vi "Format to Technique Parameter (Depreciated).vi"(0 "Potentiostat Galvanostat in":refnum<class "Potentiostat Galvanostat.lvclass">, 5 "Parameter Label":string, 7 "Parameter":variant, 9 "Parameter Index":i32, 11 "error in (no error)":errorcluster) -> (4 "Potentiostat Galvanostat out":refnum<class "Potentiostat Galvanostat.lvclass">, 8 "Technique Parameter":T1 {"Parameter Type" items=["I32 (Long)", "BOOL (Boolean)", "SGL (Single Precision)"]}, 15 "error out":errorcluster)   [LabVIEW 2018, in "Potentiostat Galvanostat.lvclass"]
doc: "This function tests the communication speed between the library and the selected channel. \nNOTE: This function is for advanced user only."
uses:
  Potentiostat Galvanostat.lvclass
  Controls/Technique Parameter.ctl
  Controls/Parameter Type.ctl
  Controls/Error Codes.ctl
  Potentiostat Galvanostat.lvclass/Potentiostat Galvanostat.ctl
  BL_GetErrorMsg.vi
  <vilib>/Utility/error.llb/Error Cluster From Error Code.vi
  <vilib>/Utility/Data Type/NI_Data Type.lvlib
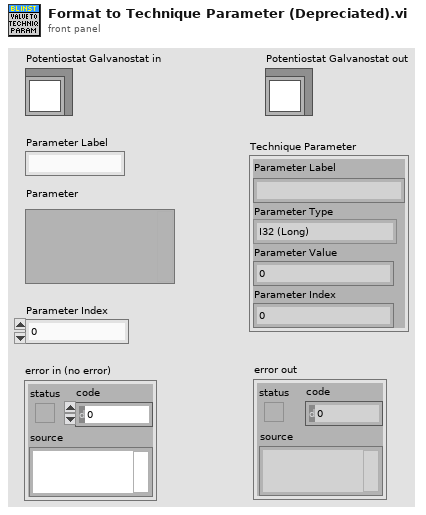
[diagram p1: front panel]
types:
  T1 = typedef "Potentiostat Galvanostat.lvclass/Technique Parameter.ctl" = cluster{"Parameter Label":string, "Parameter Type":T2, "Parameter Value":i32, "Parameter Index":i32}
  T2 = typedef "Potentiostat Galvanostat.lvclass/Parameter Type.ctl" = i32
  T3 = typedef "NI_Data Type.lvlib/Data Type.ctl" = enum8{"Invalid Type", "Void", "I8", "I16", "I32", "I64", "U8", "U16", "U32", "U64", "Single Float", "Double Float", "Extended Float", "Single Complex", "Double Complex", "Extended Complex", "Enum U8", "Enum U16", "Enum U32", "Enum U64", "Single Float With Unit", "Double Float With Unit", "Extended Float With Unit", "Single Complex with Unit", "Double Complex with Unit", "Extended Complex with Unit", "Boolean", "String", "Path", "Picture", "Tag", "Array", "Cluster", "Variant", "LV Variant", "Waveform", "Timestamp", "Digital Waveform", "Digital Data", "ExpressData", "Refnum", "External Data", "VI", "Poly VI", "LabVIEW Class Instance", "Fixed Point"}
  T4 = typedef "Potentiostat Galvanostat.lvclass/Error Codes.ctl" = i32
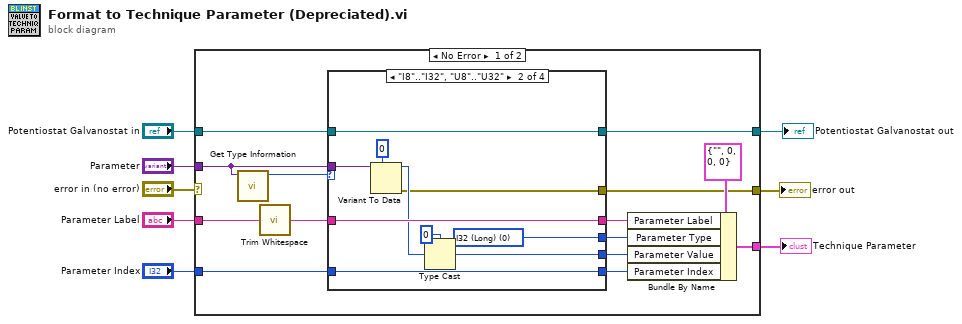
[diagram p0: block diagram]
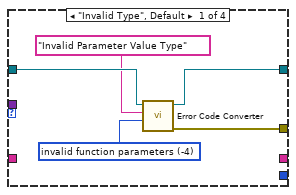
[diagram p2: hidden frame]
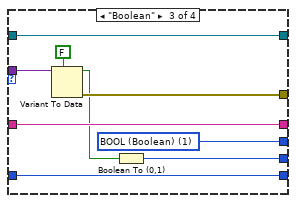
[diagram p3: hidden frame]
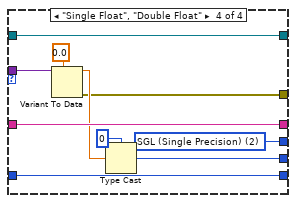
[diagram p4: hidden frame]
diagram:
  n1 = case shown="No Error" "error in (no error)" {
    selector: "error in (no error)" -> [_ w57]
    tunnel: "Parameter" -> [w10 _]
    tunnel: "Potentiostat Galvanostat in" -> [w22 w58]
    tunnel: "Parameter Label" -> [w12 _]
    tunnel: "Parameter Index" -> [w21 _]
    tunnel: [w20 _] -> w4
    tunnel: [w14 w57] -> w3
    tunnel: [w13 w58] -> w2
    frame No Error {
      n2 = call <vilib>:"Get Type Information.vi"("Variant"=w10) -> ("Type"=w9:T3)  [unwired: 6 in, 4 out]
      n3 = call <vilib>:"Trim Whitespace.vi"("string"=w12) -> ("trimmed string"=w11:string)  [unwired: 1 in]
      n4 = case shown="\"I8\"..\"I32\", \"U8\"..\"U32\"" w9 {
        tunnel: w10 -> [_ w37 w46 w56]
        tunnel: w22 -> [w27 w28 w40 w47]
        tunnel: [w26 w28 w40 w47] -> w13
        tunnel: [w25 w29 w41 w48] -> w14
        tunnel: w11 -> [_ w35 w44 w54]
        tunnel: w21 -> [_ w34 w43 w53]
        tunnel: [_ w35 w44 w54] -> w18
        tunnel: [_ w30 w42 w49] -> w17
        tunnel: [_ w33 w39 w52] -> w16
        tunnel: [_ w34 w43 w53] -> w15
        frame "Invalid Type", Default {
          w23 = T4 -4 items=["No Error"=0, "no instrument connected"=-1, "connection in progress"=-2, "selected channel(s) unplugged"=-3, "invalid function parameters"=-4, "selected file does not exist"=-5, "function failed"=-6, "no channel selected"=-7, "invalid instrument configuration"=-8, "EC-Lab firmware loaded on the instrument"=-9, "library not correctly loaded in memory"=-10, "USB library not correctly loaded in memory"=-11, "function of the library already in progress"=-12, "selected channel(s) already used"=-13, "device not allowed"=-14, "Invalid update function parameters"=-15, "internal instrument communication failed"=-101, "too many data to transfer from the instrument (device error)"=-102, "selected channel(s) unplugged (device error)"=-103, "instrument response error"=-104, "invalid message size"=-105] ("Error Code")
          n5 = call "Error Code Converter.vi"("Error Code"=w23, "Additional Description"="Invalid Parameter Value Type", "Potentiostat Galvanostat in"=w27) -> ("error out"=w25:errorcluster, "Potentiostat Galvanostat out"=w26:refnum<class "Potentiostat Galvanostat.lvclass">)  [unwired: 7 in]
        }
        frame "I8".."I32", "U8".."U32" {
          w30 = T2 0 items=["I32 (Long)", "BOOL (Boolean)", "SGL (Single Precision)"] ("Parameter Type")
          n6 = Variant To Data(type=0, Variant=w37) -> (data=w31:i32, error out=w29:errorcluster)  [unwired: 1 in]
          n7 = Type Cast(type=0, x=w31) -> (*(type *) &x=w33:i32)
        }
        frame "Boolean" {
          w42 = T2 1 items=["I32 (Long)", "BOOL (Boolean)", "SGL (Single Precision)"] ("Parameter Type")
          n8 = Variant To Data(type=FALSE, Variant=w46) -> (data=w38:bool, error out=w41:errorcluster)  [unwired: 1 in]
          n9 = Boolean To (0,1)(Boolean=w38) -> (0, 1=w39:i16)
        }
        frame "Single Float", "Double Float" {
          w49 = T2 2 items=["I32 (Long)", "BOOL (Boolean)", "SGL (Single Precision)"] ("Parameter Type")
          n10 = Variant To Data(type=sgl 0.0 ("Numeric"), Variant=w56) -> (data=w50:sgl, error out=w48:errorcluster)  [unwired: 1 in]
          n11 = Type Cast(type=0, x=w50) -> (*(type *) &x=w52:i32)
        }
      }
      n12 = Bundle By Name(cluster=T1 {"Parameter Label"="", "Parameter Type"=0, "Parameter Value"=0, "Parameter Index"=0} ("Technique Parameter"), "Parameter Label"=w18, "Parameter Type"=w17, "Parameter Value"=w16, "Parameter Index"=w15) -> (w20:T1)
    }
    frame Error {
    }
  }
  "error out" <- w3
  "Potentiostat Galvanostat out" <- w2
  "Technique Parameter" <- w4
